vi "AddText2Image.vi"(8 "error in (no error)":errorcluster, 9 "High Resolution":bool, 10 "TextOnImage":T2={"Status"="Stopped", "Experiment Name"="Experimt", "Current Temp (C)"="23.3", "Set Point (C)"="23.3", "Cooling Rate (C/min)"="x50", "Mag"=enum."20x_LM"}, 11 "Input Image":T3) -> (0 "error out":errorcluster, 3 "Output Image":T3)   [LabVIEW 2013]
doc: "Use this template to build a VI to use as a subVI."
uses:
  <vilib>/vision/Image Controls.llb/IMAQ Image.ctl
  TextOnImage.ctl
  Mag.ctl
  <vilib>/vision/NI_Vision_Development_Module.lvlib
panel:
  out "Mag":T1=enum."20x_LM"
  out "Reference Image":T3(plugin-control)
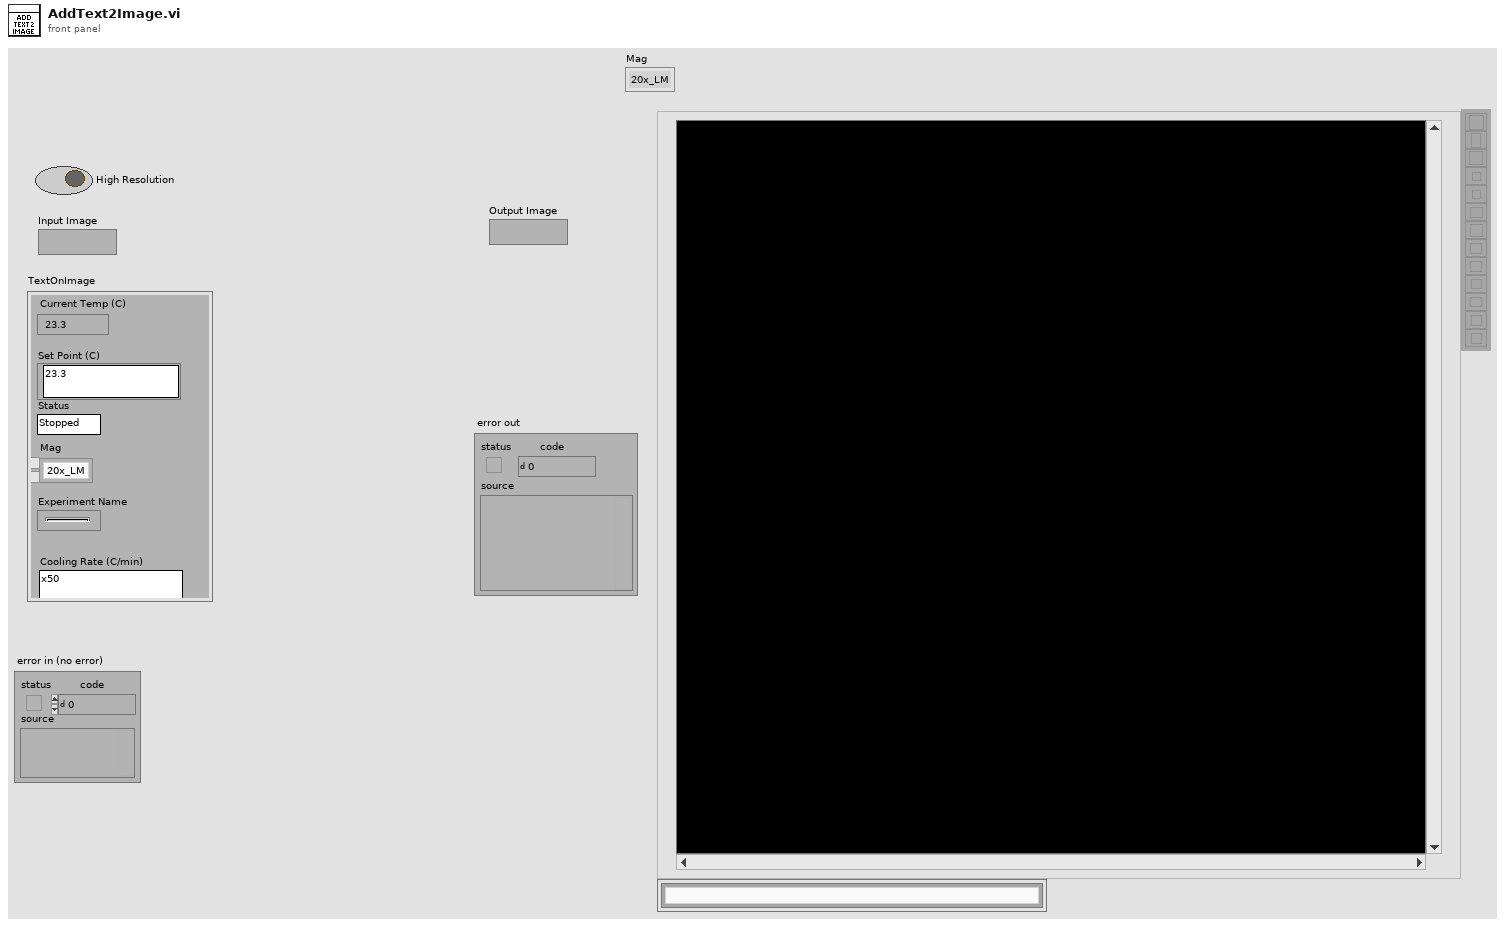
[diagram p1: front panel]
types:
  T1 = typedef "Mag.ctl" = enum16{"5x_M_BD", "10x_M", "10xM_BD", "10x_ph1", "20x_S", "20x_LM", "50x_S"}
  T2 = typedef "TextOnImage.ctl" = cluster{"Status":string, "Experiment Name":string, "Current Temp (C)":string, "Set Point (C)":string, "Cooling Rate (C/min)":string, "Mag":T1}
  T3 = typedef "IMAQ Image.ctl" = refnum<image>
  T4 = cluster{"Desired Font (Application)":enum16{"User-specified Font", "Application Font", "System Font", "Dialog Font"}, "[User-specified Font]":cluster{"Font Name":string, "Size":i16, "Strikeout?":bool, "Italic?":bool, "Underline?":bool, "Outline?":bool, "Shadow?":bool, "Bold?":bool, "Rotation Angle":dbl}, "Horizontal Alignment":i16, "Vertical Alignment":i16}
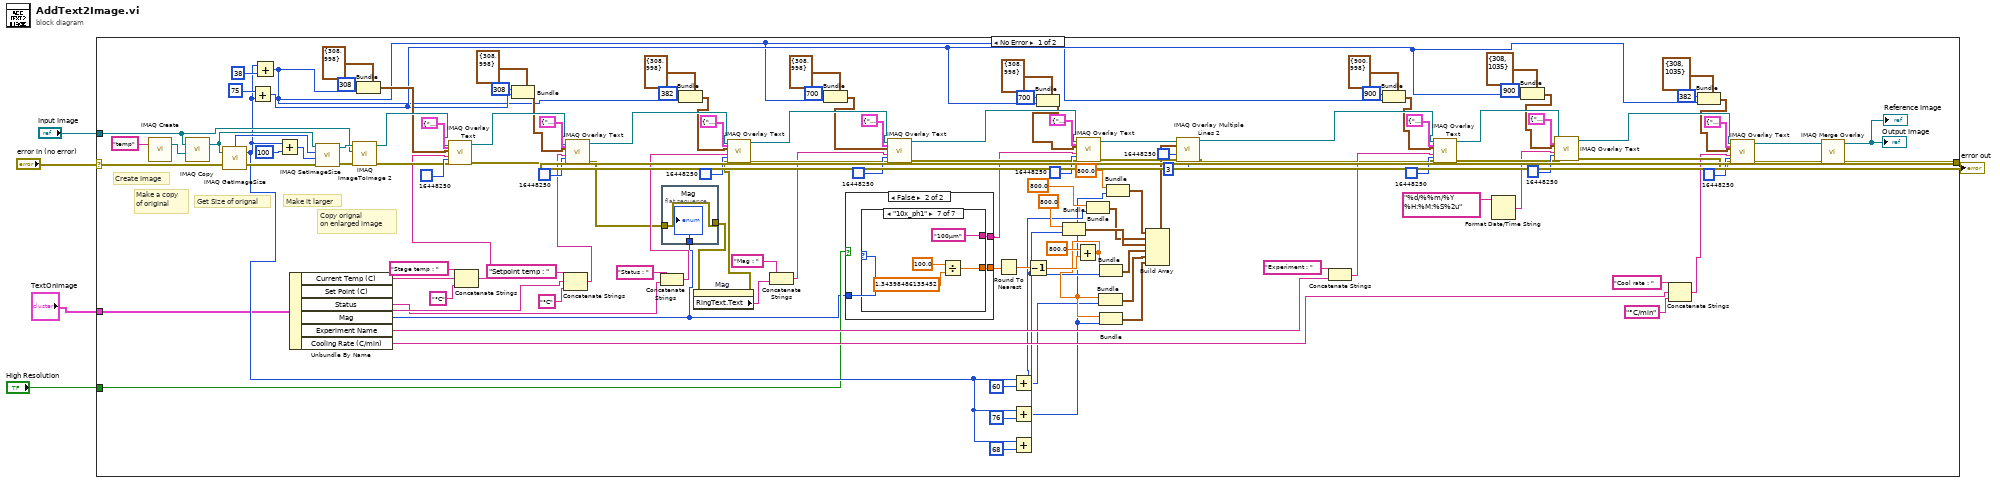
[diagram p0: block diagram]
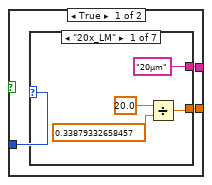
[diagram p2: hidden frame]
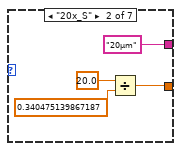
[diagram p3: hidden frame]
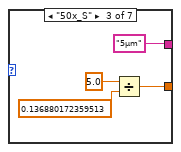
[diagram p4: hidden frame]
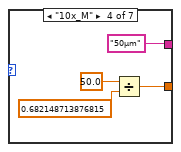
[diagram p5: hidden frame]
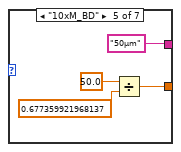
[diagram p6: hidden frame]
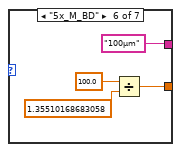
[diagram p7: hidden frame]
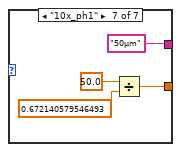
[diagram p8: hidden frame]
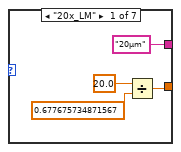
[diagram p9: hidden frame]
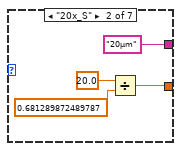
[diagram p10: hidden frame]
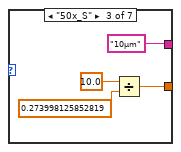
[diagram p11: hidden frame]
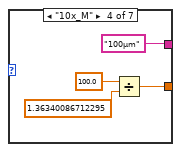
[diagram p12: hidden frame]
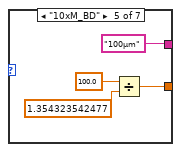
[diagram p13: hidden frame]
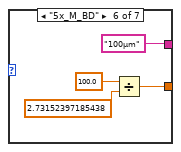
[diagram p14: hidden frame]
diagram:
  n1 = case shown="No Error" "error in (no error)" {
    selector: "error in (no error)" -> [w135 w200]
    tunnel: [w123 w200] -> w4
    tunnel: "Input Image" -> [w125 _]
    tunnel: "TextOnImage" -> [w12 _]
    tunnel: "High Resolution" -> [w11 _]
    frame No Error {
      # "Copy orignal\non enlarged image"
      # "Make it larger"
      # "Get Size of orignal"
      # "Make a copy\nof original"
      # "Create Image"
      n2 = call "IMAQ Create"("Image Name"="temp") -> ("New Image"=w127:T3)  [unwired: 4 in, 1 out]
      n3 = call "IMAQ Copy"("Image Dst"=w127, "Image Src"=w125) -> ("Image Dst Out"=w126:T3)  [unwired: 4 in, 1 out]
      n4 = call "IMAQ GetImageSize"("Image"=w126, "error in (no error)"=w135) -> ("Y Resolution"=w23:i32, "X Resolution"=w134:i32, "error out"=w133:errorcluster)  [unwired: 2 in]
      n5 = Add(x=75, y=w23) -> (x+y=w28:i32)
      n6 = Add(x=w23, y=38) -> (x+y=w26:i32)
      n7 = Add(x=w23, y=100) -> (x+y=w131:i32)
      n8 = Unbundle By Name(w12) -> ("Current Temp (C)"=w117:string, "Set Point (C)"=w108:string, "Status"=w102:string, "Mag"=w10:T1, "Experiment Name"=w91:string, "Cooling Rate (C/min)"=w75:string)
      n9 = call "IMAQ SetImageSize"("error in (no error)"=w133, "Y Resolution"=w131, "X Resolution"=w134, "Image"=w126) -> ("error out"=w128:errorcluster, "Image Out"=w129:T3)  [unwired: 1 in]
      n10 = call "IMAQ ImageToImage 2"("error in (no error)"=w128, "Image Src (Small)"=w125, "Image Src (Large)"=w129) -> ("error out"=w120:errorcluster, "Image Dst Out"=w119:T3)  [unwired: 7 in]
      n11 = Bundle(cluster=cluster{"X":i32, "Y":i32} {"X"=308, "Y"=998} ("Origin"), "X"=308, "Y"=w26) -> (w49:cluster{"X":i32, "Y":i32})
      n12 = Concatenate Strings("Stage temp : " ("string"), w117, "°C" ("string")) -> (w116:string)
      n13 = call "IMAQ Overlay Text"("Text Color (black)"=u32 16448250, "Font, Size & Style"=T4 {"Desired Font (Application)"=enum."User-specified Font", "[User-specified Font]"={"Font Name"="", "Size"=32, "Strikeout?"=FALSE, "Italic?"=FALSE, "Underline?"=FALSE, "Outline?"=FALSE, "Shadow?"=FALSE, "Bold?"=TRUE, "Rotation Angle"=0.0}, "Horizontal Alignment"=2, "Vertical Alignment"=2}, "error in (no error)"=w120, "String"=w116, "Origin"=w49, "Image"=w119) -> ("error out"=w111:errorcluster, "Image Out"=w112:T3)  [unwired: 4 in]
      n14 = Bundle(cluster=cluster{"X":i32, "Y":i32} {"X"=308, "Y"=998} ("Origin"), "X"=308, "Y"=w28) -> (w31:cluster{"X":i32, "Y":i32})
      n15 = Concatenate Strings("Setpoint temp : " ("string"), w108, "°C" ("string")) -> (w107:string)
      n16 = call "IMAQ Overlay Text"("Text Color (black)"=u32 16448250, "Font, Size & Style"=T4 {"Desired Font (Application)"=enum."User-specified Font", "[User-specified Font]"={"Font Name"="", "Size"=32, "Strikeout?"=FALSE, "Italic?"=FALSE, "Underline?"=FALSE, "Outline?"=FALSE, "Shadow?"=FALSE, "Bold?"=TRUE, "Rotation Angle"=0.0}, "Horizontal Alignment"=2, "Vertical Alignment"=2}, "error in (no error)"=w111, "String"=w107, "Origin"=w31, "Image"=w112) -> ("error out"=w7:errorcluster, "Image Out"=w104:T3)  [unwired: 4 in]
      n17 = Concatenate Strings("Status : " ("string"), w102) -> (w101:string)
      n18 = flat-sequence {
        tunnel: w10 -> [w137]
        tunnel: [w136] -> w8
        tunnel: w7 -> [w136]
        frame #0 {
          "Mag" <- w137
        }
      }
      n19 = Bundle(cluster=cluster{"X":i32, "Y":i32} {"X"=308, "Y"=998} ("Origin"), "X"=382, "Y"=w26) -> (w42:cluster{"X":i32, "Y":i32})
      n20 = property on="Mag" class="Enum (strict)"(error in=w8) -> (error out=w6:errorcluster, "RingText.Text"=w9:string)  [unwired: 1 in, 1 out]
      n21 = call "IMAQ Overlay Text"("Text Color (black)"=u32 16448250, "Font, Size & Style"=T4 {"Desired Font (Application)"=enum."User-specified Font", "[User-specified Font]"={"Font Name"="", "Size"=32, "Strikeout?"=FALSE, "Italic?"=FALSE, "Underline?"=FALSE, "Outline?"=FALSE, "Shadow?"=FALSE, "Bold?"=TRUE, "Rotation Angle"=0.0}, "Horizontal Alignment"=0, "Vertical Alignment"=2}, "error in (no error)"=w6, "String"=w101, "Origin"=w42, "Image"=w104) -> ("error out"=w97:errorcluster, "Image Out"=w98:T3)  [unwired: 4 in]
      n22 = Concatenate Strings("Mag : " ("string"), w9) -> (w95:string)
      n23 = Bundle(cluster=cluster{"X":i32, "Y":i32} {"X"=308, "Y"=998} ("Origin"), "X"=700, "Y"=w26) -> (w41:cluster{"X":i32, "Y":i32})
      n24 = case shown="False" w11 {
        tunnel: w10 -> [w140 w171]
        tunnel: [w139 w170] -> w63
        tunnel: [w138 w169] -> w60
        frame True {
          n25 = case shown="\"20x_LM\"" w140 {
            tunnel: [w142 w146 w150 w154 w158 w162 w166] -> w139
            tunnel: ["20µm" ("string") "20µm" ("string") "5µm" ("string") "50µm" ("string") "50µm" ("string") "100µm" ("string") "50µm" ("string")] -> w138
            frame "20x_LM" {
              n26 = Divide(x=20.0, y=0.33879332658457) -> (x/y=w142:dbl)
            }
            frame "20x_S" {
              n27 = Divide(x=20.0, y=0.340475139867187) -> (x/y=w146:dbl)
            }
            frame "50x_S" {
              n28 = Divide(x=5.0, y=0.136880172359513) -> (x/y=w150:dbl)
            }
            frame "10x_M" {
              n29 = Divide(x=50.0, y=0.682148713876815) -> (x/y=w154:dbl)
            }
            frame "10xM_BD" {
              n30 = Divide(x=50.0, y=0.677359921968137) -> (x/y=w158:dbl)
            }
            frame "5x_M_BD" {
              n31 = Divide(x=100.0, y=1.35510168683058) -> (x/y=w162:dbl)
            }
            frame "10x_ph1" {
              n32 = Divide(x=50.0, y=0.672140579546493) -> (x/y=w166:dbl)
            }
          }
        }
        frame False {
          n33 = case shown="\"10x_ph1\"" w171 {
            tunnel: [w173 w177 w181 w185 w189 w193 w197] -> w170
            tunnel: ["20µm" ("string") "20µm" ("string") "10µm" ("string") "100µm" ("string") "100µm" ("string") "100µm" ("string") "100µm" ("string")] -> w169
            frame "20x_LM" {
              n34 = Divide(x=20.0, y=0.677675734871567) -> (x/y=w173:dbl)
            }
            frame "20x_S" {
              n35 = Divide(x=20.0, y=0.681289872489787) -> (x/y=w177:dbl)
            }
            frame "50x_S" {
              n36 = Divide(x=10.0, y=0.273998125852819) -> (x/y=w181:dbl)
            }
            frame "10x_M" {
              n37 = Divide(x=100.0, y=1.36340086712295) -> (x/y=w185:dbl)
            }
            frame "10xM_BD" {
              n38 = Divide(x=100.0, y=1.354323542477) -> (x/y=w189:dbl)
            }
            frame "5x_M_BD" {
              n39 = Divide(x=100.0, y=2.73152397185438) -> (x/y=w193:dbl)
            }
            frame "10x_ph1" {
              n40 = Divide(x=100.0, y=1.34398486135452) -> (x/y=w197:dbl)
            }
          }
        }
      }
      n41 = call "IMAQ Overlay Text"("Text Color (black)"=u32 16448250, "Font, Size & Style"=T4 {"Desired Font (Application)"=enum."User-specified Font", "[User-specified Font]"={"Font Name"="", "Size"=32, "Strikeout?"=FALSE, "Italic?"=FALSE, "Underline?"=FALSE, "Outline?"=FALSE, "Shadow?"=FALSE, "Bold?"=TRUE, "Rotation Angle"=0.0}, "Horizontal Alignment"=0, "Vertical Alignment"=2}, "error in (no error)"=w97, "String"=w95, "Origin"=w41, "Image"=w98) -> ("error out"=w70:errorcluster, "Image Out"=w71:T3)  [unwired: 4 in]
      n42 = Round To Nearest(number=w63) -> (nearest integer value=w62:dbl)
      n43 = Add(x=w23, y=60) -> (x+y=w17:i32)
      n44 = Add(x=w23, y=76) -> (x+y=w13:i32)
      n45 = Add(x=w23, y=68) -> (x+y=w21:i32)
      n46 = Decrement(x=w62) -> (x-1=w61:dbl)
      n47 = Bundle(cluster=cluster{"X":i32, "Y":i32} {"X"=308, "Y"=998} ("Origin"), "X"=700, "Y"=w28) -> (w30:cluster{"X":i32, "Y":i32})
      n48 = Bundle("x"=800.0, w21) -> (w19:cluster{"x":dbl, i32})  [unwired: 1 in]
      n49 = Add(x=800.0, y=w61) -> (x+y=w57:dbl)
      n50 = call "IMAQ Overlay Text"("Text Color (black)"=u32 16448250, "Font, Size & Style"=T4 {"Desired Font (Application)"=enum."User-specified Font", "[User-specified Font]"={"Font Name"="", "Size"=32, "Strikeout?"=FALSE, "Italic?"=FALSE, "Underline?"=FALSE, "Outline?"=FALSE, "Shadow?"=FALSE, "Bold?"=TRUE, "Rotation Angle"=0.0}, "Horizontal Alignment"=0, "Vertical Alignment"=2}, "error in (no error)"=w70, "String"=w60, "Origin"=w30, "Image"=w71) -> ("error out"=w69:errorcluster, "Image Out"=w68:T3)  [unwired: 4 in]
      n51 = Bundle("x"=800.0, w17) -> (w16:cluster{"x":dbl, i32})  [unwired: 1 in]
      n52 = Bundle(w57, w17) -> (w56:cluster{dbl, i32})  [unwired: 1 in]
      n53 = Bundle(w57, w21) -> (w59:cluster{dbl, i32})  [unwired: 1 in]
      n54 = Bundle(w57, w13) -> (w55:cluster{dbl, i32})  [unwired: 1 in]
      n55 = Bundle("x"=800.0, w13) -> (w14:cluster{"x":dbl, i32})  [unwired: 1 in]
      n56 = Build Array(w14, w16, w19, w59, w56, w55) -> (w65:cluster{"x":dbl, i32}[])
      n57 = call "IMAQ Overlay Multiple Lines 2"("Image"=w68, "Line End Points"=w65, "Color"=u32 16448250, "error in (no error)"=w69, "Width"=u32 3) -> ("Image Out"=w67:T3, "error out"=w66:errorcluster)  [unwired: 9 in]
      n58 = Concatenate Strings("Experiment : " ("string"), w91) -> (w90:string)
      n59 = Bundle(cluster=cluster{"X":i32, "Y":i32} {"X"=900, "Y"=998} ("Origin"), "X"=900, "Y"=w26) -> (w40:cluster{"X":i32, "Y":i32})
      n60 = call "IMAQ Overlay Text"("Text Color (black)"=u32 16448250, "Font, Size & Style"=T4 {"Desired Font (Application)"=enum."User-specified Font", "[User-specified Font]"={"Font Name"="", "Size"=32, "Strikeout?"=FALSE, "Italic?"=FALSE, "Underline?"=FALSE, "Outline?"=FALSE, "Shadow?"=FALSE, "Bold?"=TRUE, "Rotation Angle"=0.0}, "Horizontal Alignment"=0, "Vertical Alignment"=2}, "error in (no error)"=w66, "String"=w90, "Origin"=w40, "Image"=w67) -> ("error out"=w86:errorcluster, "Image Out"=w87:T3)  [unwired: 4 in]
      n61 = Format Date/Time String(time format string (%c)="%d/%%m/%Y %H:%M:%S%2u") -> (date/time string=w84:string)  [unwired: 2 in]
      n62 = Bundle(cluster=cluster{"X":i32, "Y":i32} {"X"=308, "Y"=1035} ("Origin"), "X"=900, "Y"=w28) -> (w29:cluster{"X":i32, "Y":i32})
      n63 = call "IMAQ Overlay Text"("Text Color (black)"=u32 16448250, "Font, Size & Style"=T4 {"Desired Font (Application)"=enum."User-specified Font", "[User-specified Font]"={"Font Name"="", "Size"=32, "Strikeout?"=FALSE, "Italic?"=FALSE, "Underline?"=FALSE, "Outline?"=FALSE, "Shadow?"=FALSE, "Bold?"=TRUE, "Rotation Angle"=0.0}, "Horizontal Alignment"=0, "Vertical Alignment"=2}, "error in (no error)"=w86, "String"=w84, "Origin"=w29, "Image"=w87) -> ("error out"=w80:errorcluster, "Image Out"=w81:T3)  [unwired: 4 in]
      n64 = Concatenate Strings("Cool rate : " ("string"), w75, "°C/min" ("string")) -> (w74:string)
      n65 = Bundle(cluster=cluster{"X":i32, "Y":i32} {"X"=308, "Y"=1035} ("Origin"), "X"=382, "Y"=w28) -> (w27:cluster{"X":i32, "Y":i32})
      n66 = call "IMAQ Overlay Text"("Text Color (black)"=u32 16448250, "Font, Size & Style"=T4 {"Desired Font (Application)"=enum."User-specified Font", "[User-specified Font]"={"Font Name"="", "Size"=32, "Strikeout?"=FALSE, "Italic?"=FALSE, "Underline?"=FALSE, "Outline?"=FALSE, "Shadow?"=FALSE, "Bold?"=TRUE, "Rotation Angle"=0.0}, "Horizontal Alignment"=0, "Vertical Alignment"=2}, "error in (no error)"=w80, "String"=w74, "Origin"=w27, "Image"=w81) -> ("error out"=w78:errorcluster, "Image Out"=w79:T3)  [unwired: 4 in]
      n67 = call "IMAQ Merge Overlay"("error in (no error)"=w78, "Image Src"=w79) -> ("error out"=w123:errorcluster, "Image Dst Out"=→"Output Image" →"Reference Image":T3)  [unwired: 8 in]
    }
    frame Error {
    }
  }
  "error out" <- w4
